vi "WindToSailLookupTest-OLD.vi"() -> (3 "Were there any errors at all?":bool)   [LabVIEW 2013]
panel:
  out "Are Jib Suggestions Right?":bool[](array[boolean])=[TRUE, TRUE, TRUE, TRUE, TRUE, TRUE]
  out "Are Main Suggestion Right?":bool[](array[boolean])=[TRUE, TRUE, TRUE, TRUE, TRUE, TRUE]
  out "Actual Jib Sail Suggestions":dbl[](array[numeric])=[0.0, 0.0, 1.0, 0.5, 1.0, 0.0]
  out "Actual Main Sail Suggestions":dbl[](array[numeric])=[0.0, 0.0, 1.0, 0.5, 1.0, 0.0]
  in  "Expected Jib Outputs":dbl[](array[numeric])=[0.0, 0.0, 1.0, 0.5, 1.0, 0.0]
  in  "Expected Main Outputs":dbl[](array[numeric])=[0.0, 0.0, 1.0, 0.5, 1.0, 0.0]
  in  "Inputs":dbl[](array[numeric])=[0.0, 44.0, 170.0, 65.7, 300.0, -10.0]
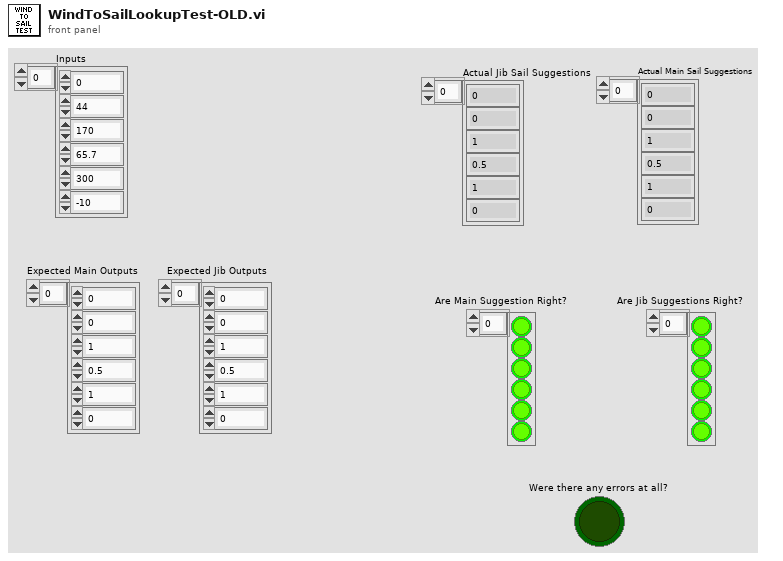
[diagram p1: front panel]
types:
  T1 = typedef "Sail Set Suggestions.ctl" = cluster{"MainSailSuggestion":dbl, "JibSailSuggestion":dbl}
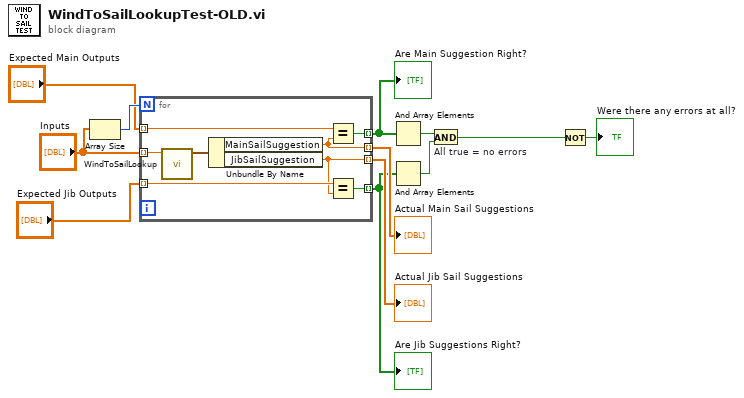
[diagram p0: block diagram]
diagram:
  n1 = Array Size(array="Inputs") -> (size(s)=w12:i32)
  n2 = for {
    N: w12 -> [_]
    tunnel: "Inputs" -> [w14] mode=indexing
    tunnel: "Expected Main Outputs" -> [w20] mode=indexing
    tunnel: "Expected Jib Outputs" -> [w19] mode=indexing
    tunnel: [w18] -> w8 mode=indexing
    tunnel: [w17] -> w7 mode=indexing
    tunnel: [w16] -> w4 mode=indexing
    tunnel: [w15] -> w6 mode=indexing
    n3 = call "WindToSailLookup.vi"("ApparentWindAngle"=w14) -> ("Suggested Sail Setpoints"=w13:T1)  [unwired: 10 in]
    n4 = Unbundle By Name(w13) -> ("MainSailSuggestion"=w18:dbl, "JibSailSuggestion"=w17:dbl)
    n5 = Equal?(x=w20, y=w18) -> (x = y?=w16:bool)
    n6 = Equal?(x=w19, y=w17) -> (x = y?=w15:bool)
  }
  "Actual Main Sail Suggestions" <- w8
  "Actual Jib Sail Suggestions" <- w7
  "Are Main Suggestion Right?" <- w4
  "Are Jib Suggestions Right?" <- w6
  n7 = And Array Elements(Boolean array=w4) -> (logical AND=w3:bool)
  n8 = And Array Elements(Boolean array=w6) -> (logical AND=w5:bool)
  n9 = And "All true = no errors"(x=w3, y=w5) -> (x .and. y?=w2:bool)
  n10 = Not(x=w2) -> (.not. x?=→"Were there any errors at all?":bool)
